vi "TempControllerMain_11.vi"() -> ()   [LabVIEW 2012]
uses:
  Controls/stateEnum.ctl
  Controls/FGV Function.ctl
panel:
  out "Heating":bool
  in  "Calibrate":bool
  out "1st":i32
  out "2nd":i32
  in  "Set Point":dbl
  in  "Mode":bool
  out "Current Temperature":dbl
  in  "Stop Button":bool
  in  "Save Directory":path
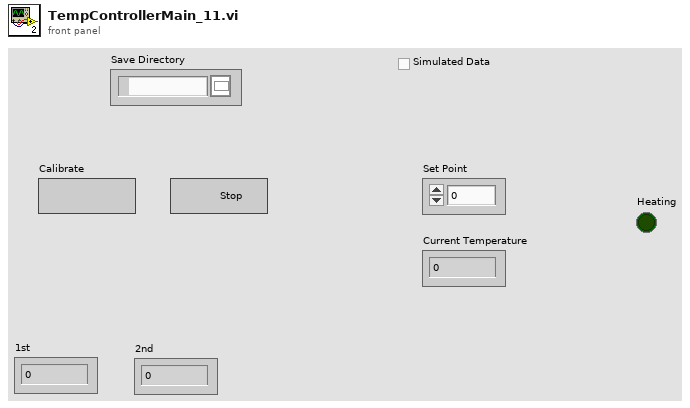
[diagram p1: front panel]
types:
  T1 = typedef "FGV Function.ctl" = enum16{"Initiate", "Read", "Set On", "Set Off"}
  T2 = typedef "stateEnum.ctl" = enum16{"Initialise", "Set Voltage On", "Set Voltage Off"}
  T3 = cluster{"Save Path":path, "Set Point":dbl, "Current Temperature":dbl, "Stop Button Pressed?":bool, "States":T2}
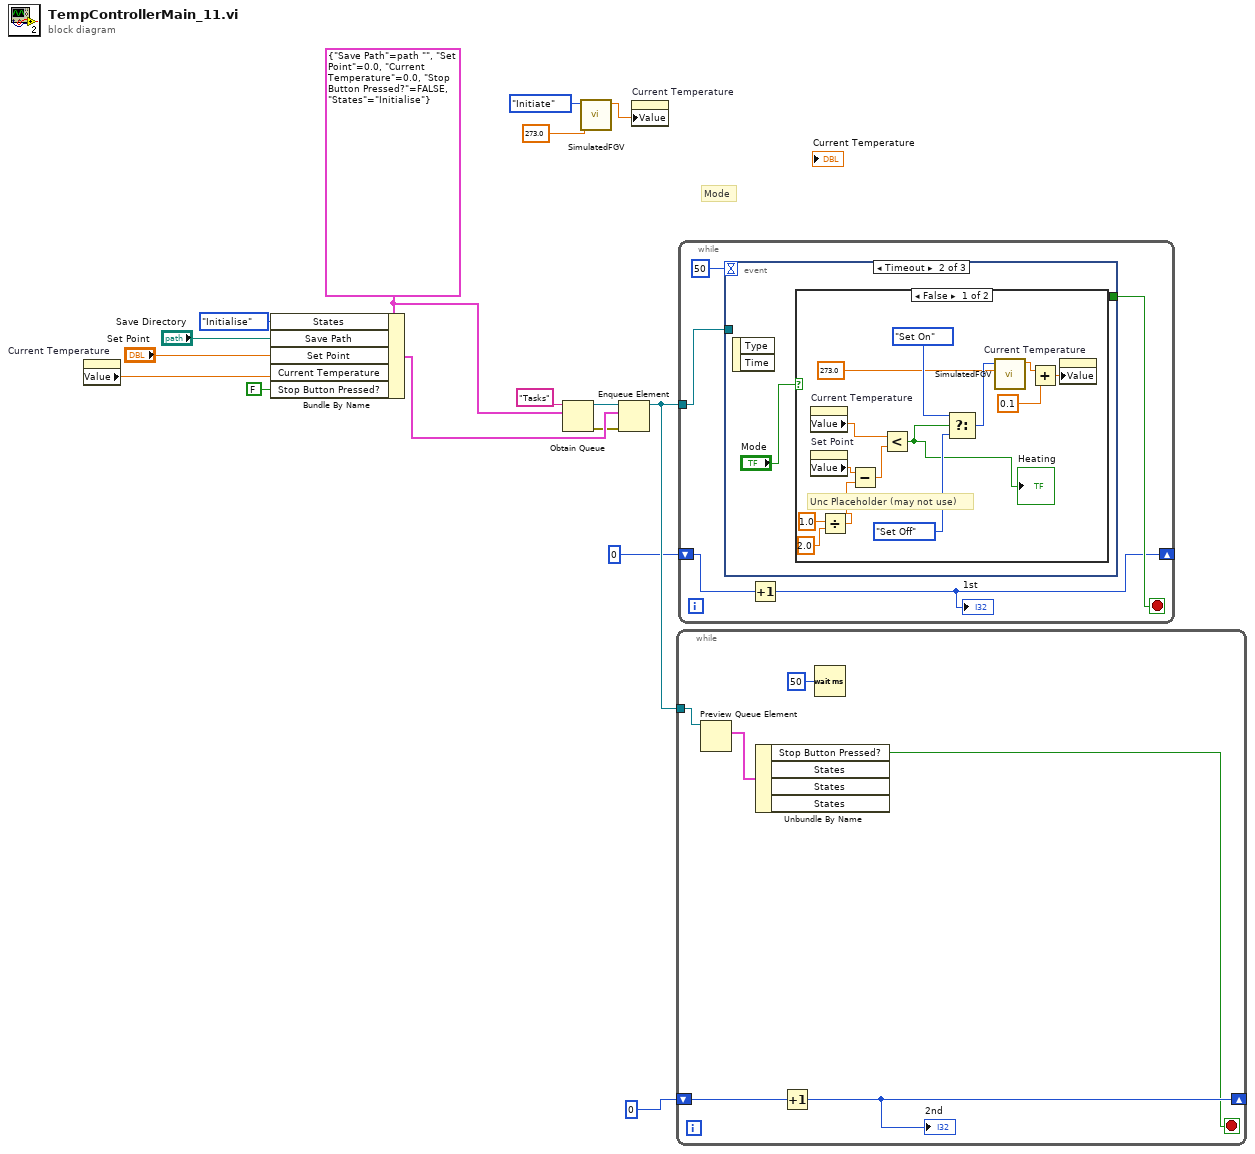
[diagram p0: block diagram]
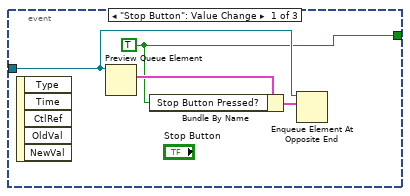
[diagram p2: hidden frame]
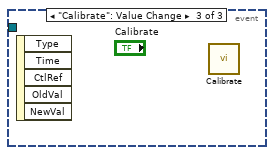
[diagram p4: hidden frame]
diagram:
  w10 = T3 {"Save Path"=path "", "Set Point"=0.0, "Current Temperature"=0.0, "Stop Button Pressed?"=FALSE, "States"=enum."Initialise"}
  # "Mode"
  n1 = property on="Current Temperature" class="DigNum (strict)"() -> ("Value"=w12:dbl)  [unwired: 2 in, 2 out]
  n2 = Bundle By Name(cluster=w10, "States"=stateEnum."Initialise", "Save Path"="Save Directory", "Set Point"="Set Point", "Current Temperature"=w12, "Stop Button Pressed?"=FALSE) -> (w8:T3)
  n3 = Obtain Queue(name (unnamed)="Tasks", element data type=w10) -> (queue out=w9:refnum<queue>, error out=w7:errorcluster)  [unwired: 3 in, 1 out]
  n4 = call "SimulatedFGV.vi"("Starting Temperature"=273.0, "FGV Function"=FGV_Function."Initiate") -> ("Current Temperature"=w3:dbl)  [unwired: 9 in]
  n5 = Enqueue Element(queue=w9, element=w8, error in (no error)=w7) -> (queue out=w5:refnum<queue>)  [unwired: 1 in, 2 out]
  n6 = property on="Current Temperature" class="DigNum (strict)"("Value"=w3) -> ()  [unwired: 2 in, 2 out]
  n7 = while {
    shift-right: [w21] -> _
    shift-left: 0 -> [w22]
    tunnel: w5 -> [w18]
    stop <- w19 stop-if-true
    n8 = Preview Queue Element(queue=w18) -> (element=w17:T3)  [unwired: 2 in, 3 out]
    n9 = Unbundle By Name(w17) -> ("Stop Button Pressed?"=w19:bool)  [unwired: 3 out]
    n10 = Increment(x=w22) -> (x+1=w21:i32)
    "2nd" <- w21
    n11 = Wait (ms)(milliseconds to wait=u32 50) -> ()  [unwired: 1 out]
  }
  n12 = while {
    tunnel: w5 -> [w27]
    shift-right: [w24] -> _
    shift-left: 0 -> [w25]
    stop <- w26 stop-if-true
    n13 = event shown="[1] Timeout" {
      selector: _ -> [_ _ _]
      dyn-events: _ -> [_ _ _]
      timeout: 50 -> [_ _ _]
      tunnel: w27 -> [w31 _ _]
      tunnel: [w28 _ _] -> w26
      event "Stop Button": Value Change {
        w28 = TRUE ("Stop Button Pressed?")
        n14 = event-data() -> ()  [unwired: 1 in, 5 out]
        n15 = Preview Queue Element(queue=w31) -> (element=w30:T3)  [unwired: 2 in, 3 out]
        n16 = Bundle By Name(cluster=w30, "Stop Button Pressed?"=w28) -> (w29:T3)
        n17 = Enqueue Element At Opposite End(queue=w31, element=w29) -> ()  [unwired: 2 in, 3 out]
      }
      event Timeout {
        n18 = event-data() -> ()  [unwired: 1 in, 2 out]
        n19 = case shown="False" "Mode" {
          frame False {
            # "Unc Placeholder (may not use)"
            n20 = property on="Current Temperature" class="DigNum (strict)"() -> ("Value"=w39:dbl)  [unwired: 2 in, 2 out]
            n21 = property on="Set Point" class="DigNum (strict)"() -> ("Value"=w37:dbl)  [unwired: 2 in, 2 out]
            n22 = Divide(x=1.0 ("y"), y=2.0) -> (x/y=w34:dbl)
            n23 = Subtract(x=w37, y=w34) -> (x-y=w36:dbl)
            n24 = Less?(x=w39, y=w36) -> (x < y?=w38:bool)
            "Heating" <- w38
            n25 = Select(t=FGV_Function."Set On" ("FGV Function"), s=w38, f=FGV_Function."Set Off" ("FGV Function")) -> (s? t:f=w44:T1)
            n26 = call "SimulatedFGV.vi"("Starting Temperature"=273.0, "FGV Function"=w44) -> ("Current Temperature"=w42:dbl)  [unwired: 9 in]
            n27 = Add(x=w42, y=0.1) -> (x+y=w41:dbl)
            n28 = property on="Current Temperature" class="DigNum (strict)"("Value"=w41) -> ()  [unwired: 2 in, 2 out]
          }
          frame True {
          }
        }
      }
      event "Calibrate": Value Change {
        n29 = event-data() -> ()  [unwired: 1 in, 5 out]
        n30 = call "Calibrate.vi"() -> ()  [unwired: 8 in, 4 out]
      }
    }
    n31 = Increment(x=w25) -> (x+1=w24:i32)
    "1st" <- w24
  }
